vi "Acionamento motor.vi"() -> ()   [LabVIEW 2020]
uses:
  <vilib>/Instr/_visa.llb/VISA Configure Serial Port (Instr).vi
panel:
  in  "OK Button":bool
  in  "stop":bool
  in  "VISA resource name":refnum<visa-resource-name>
  out "SAÍDA":string
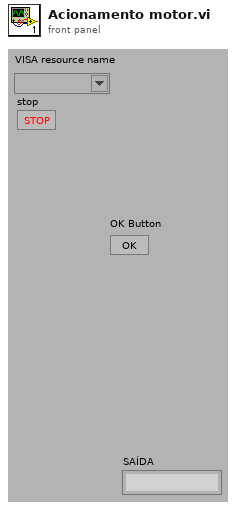
[diagram p1: front panel]
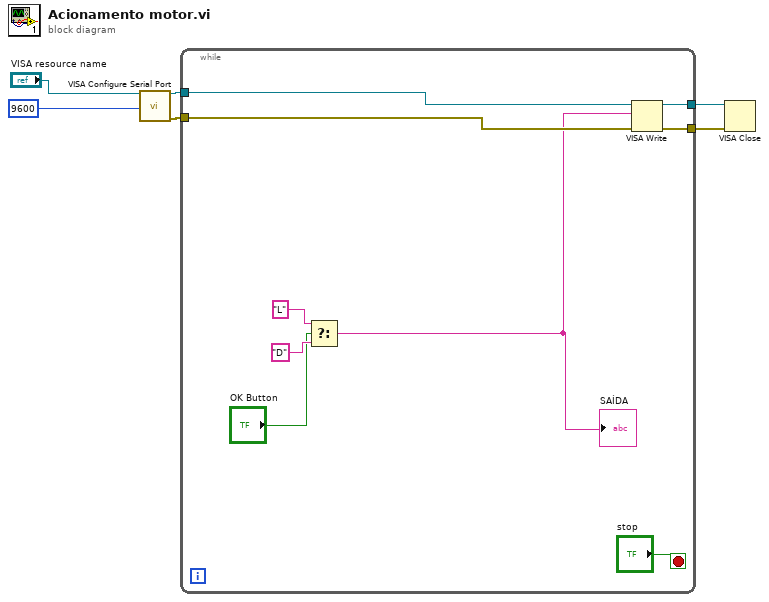
[diagram p0: block diagram]
diagram:
  n1 = call-poly "VISA Configure Serial Port"("VISA resource name"="VISA resource name", "baud rate (9600)"=u32 9600) -> ("VISA resource name out"=w5:refnum<visa-resource-name>, "error out"=w4:errorcluster)  [unwired: 12 in]
  n2 = while {
    tunnel: w5 -> [w13]
    tunnel: w4 -> [w12]
    tunnel: [w11] -> w3
    tunnel: [w10] -> w2
    stop <- "stop" stop-if-true
    n3 = Select(t="L", s="OK Button", f="D") -> (s? t:f=w8:string)
    "SAÍDA" <- w8
    n4 = VISA Write(VISA resource name=w13, write buffer=w8, error in (no error)=w12) -> (VISA resource name out=w11:refnum<visa-resource-name>, error out=w10:errorcluster)  [unwired: 1 out]
  }
  n5 = VISA Close(VISA resource name=w3, error in (no error)=w2) -> ()  [unwired: 1 out]
